vi "获取URL下载链接.vi"(8 "error in (no error)":errorcluster, 11 "固件升级":enum16{"无", "CODMn", "氨氮", "总磷", "总氮", "CODCr"}(ring)) -> (0 "error out":errorcluster, 3 "String/Binary data":string caption="URL")   [LabVIEW 2016, in "数据传输系统.lvlib" / "update.lvlib" / "http client.lvclass"]
uses:
  http client.lvclass
  <vilib>/registry/registry.llb/Registry RtKey.ctl
  <vilib>/registry/registry.llb/Read Registry Value Simple STR.vi
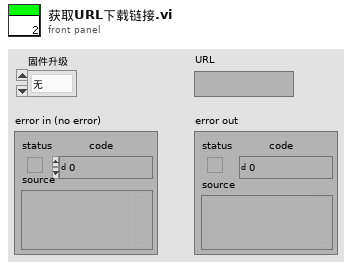
[diagram p1: front panel]
types:
  T1 = typedef "Registry RtKey.ctl" = enum32{"HKEY_CLASSES_ROOT", "HKEY_CURRENT_USER", "HKEY_LOCAL_MACHINE", "HKEY_USERS", "HKEY_PERFORMANCE_DATA", "HKEY_CURRENT_CONFIG", "HKEY_DYN_DATA"}
  T2 = typedef "Registry refnum.ctl" = refnum<k1>
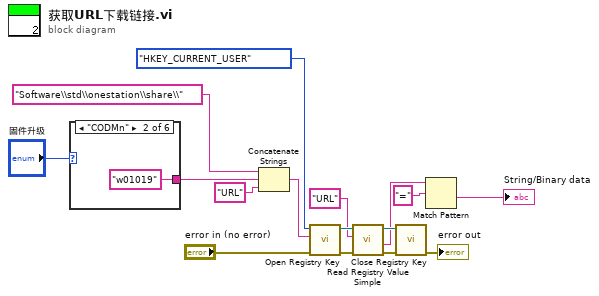
[diagram p0: block diagram]
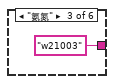
[diagram p3: hidden frame]
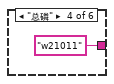
[diagram p4: hidden frame]
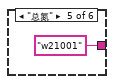
[diagram p5: hidden frame]
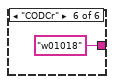
[diagram p6: hidden frame]
diagram:
  n1 = case shown="\"CODMn\"" "固件升级" {
    tunnel: [_ "w01019" "w21003" "w21011" "w21001" "w01018"] -> w2
    frame "无", Default {
    }
    frame "CODMn" {
    }
    frame "氨氮" {
    }
    frame "总磷" {
    }
    frame "总氮" {
    }
    frame "CODCr" {
    }
  }
  n2 = Concatenate Strings("Software\\std\\onestation\\share\\" ("subkey"), w2, "URL" ("URL")) -> (w3:string)
  n3 = call <vilib>:"Open Registry Key.vi"("error in (no error)"="error in (no error)", "subkey"=w3, "root key (HKEY_LOCAL_MACHINE)"=Registry_RtKey."HKEY_CURRENT_USER") -> ("error out"=w15:errorcluster, "refnum out"=w16:T2)  [unwired: 7 in]
  n4 = call-poly <vilib>:"Read Registry Value Simple.vi"("error in (no error)"=w15, "value"="URL", "refnum"=w16) -> ("error out"=w11:errorcluster, "String/Binary data"=w9:string, "refnum out"=w12:T2)  [unwired: 3 in, 1 out]
  n5 = call <vilib>:"Close Registry Key.vi"("error in (no error)"=w11, "refnum"=w12) -> ("error out"=→"error out":errorcluster)  [unwired: 5 in]
  n6 = Match Pattern(string=w9, regular expression="=" ("正则表达式")) -> (after substring=→"String/Binary data":string)  [unwired: 1 in, 3 out]
